vi "elapsed_time_randomico.vi"() -> ()   [LabVIEW 2020]
panel:
  out "Numero de iteraciones":i32
  out "number (0 to 1)":dbl
  in  "stop":bool
  out "Elapsed Time (s)":dbl
  out "Time has Elapsed":bool
  in  "Auto Reset":bool=TRUE
  in  "Reset":bool
  in  "Time Target (s)":dbl=10.0
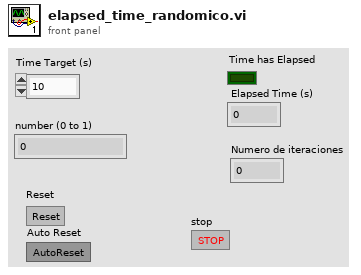
[diagram p1: front panel]
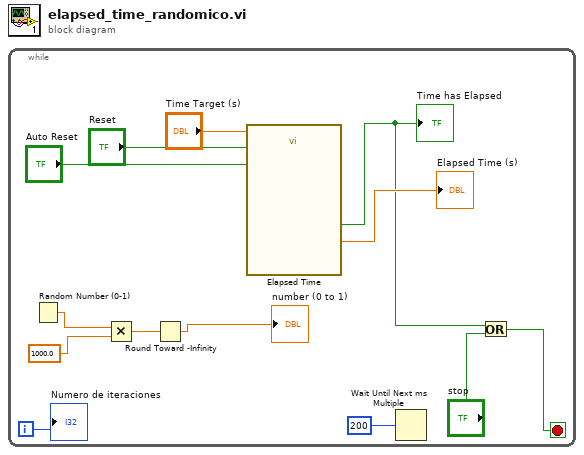
[diagram p0: block diagram]
diagram:
  n1 = while {
    i -> [w4]
    stop <- w1 stop-if-true
    n2 = Random Number (0-1)() -> (number: 0 to 1=w8:dbl)
    n3 = Multiply(x=w8, y=1000.0 ("number (0 to 1)")) -> (x*y=w7:dbl)
    n4 = Round Toward -Infinity(1:w7) -> (0:→"number (0 to 1)":dbl)
    n5 = call "Elapsed Time"("Time Target (s)"="Time Target (s)", "Reset"="Reset", "Auto Reset"="Auto Reset") -> ("Elapsed Time (s)"=→"Elapsed Time (s)":dbl, "Time has Elapsed"=w3:bool)  [unwired: 9 in, 6 out]
    "Time has Elapsed" <- w3
    n6 = Wait Until Next ms Multiple(millisecond multiple=u32 200 ("millisecond timer value")) -> ()  [unwired: 1 out]
    n7 = Or(x=w3, y="stop") -> (x .or. y?=w1:bool)
    "Numero de iteraciones" <- w4
  }
